vi "try phidget servo.vi"() -> ()   [LabVIEW 2014]
panel:
  in  "Y pos":dbl(slide)=136.3265306122449 scale=120.0..180.0
  out "error out":errorcluster
  in  "X pos":dbl(slide)=107.31292517006803 step=0.1 scale=80.0..135.0 scale format="%#.2g"
  in  "stop":bool
  out "Serial Number Return":i32
  out "Engaged?":bool
  out "Number of\nservos":i32
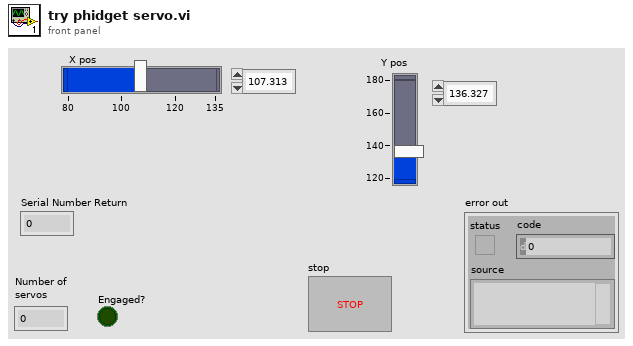
[diagram p1: front panel]
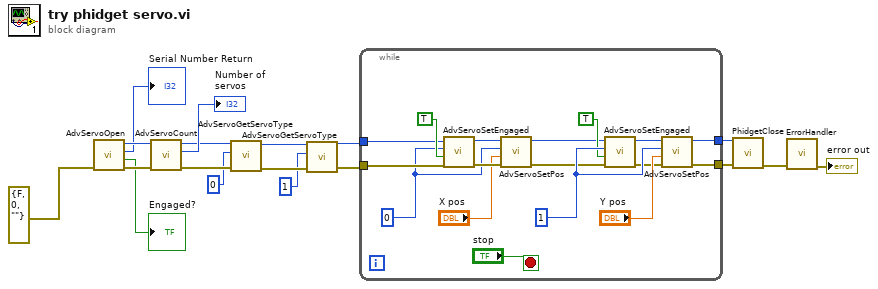
[diagram p0: block diagram]
diagram:
  n1 = call "AdvServoOpen.vi"("error in"=errorcluster {"status"=FALSE, "code"=0, "source"=""} ("error in (no error)")) -> ("error out"=w17:errorcluster, "Attached?"=→"Engaged?":bool, "Serial Number Return"=→"Serial Number Return":i32, "Device Out"=w16:i32)  [unwired: 7 in]
  n2 = call "AdvServoCount.vi"("error in (no error)"=w17, "Device In"=w16) -> ("error out"=w7:errorcluster, "count"=→"Number of\nservos":i32, "Device Out"=w8:i32)  [unwired: 7 in]
  n3 = call "AdvServoGetServoType.vi"("error in (no error)"=w7, "index"=0, "Device In"=w8) -> ("error out"=w4:errorcluster, "Device Out"=w5:i32)  [unwired: 5 in, 1 out]
  n4 = call "AdvServoGetServoType.vi"("error in (no error)"=w4, "index"=1, "Device In"=w5) -> ("error out"=w1:errorcluster, "Device Out"=w2:i32)  [unwired: 5 in, 1 out]
  n5 = while {
    tunnel: w2 -> [w32]
    tunnel: w1 -> [w31]
    tunnel: [w20] -> w10
    tunnel: [w19] -> w9
    stop <- "stop" stop-if-true
    w27 = 1
    w28 = 0
    n6 = call "AdvServoSetEngaged.vi"("error in (no error)"=w31, "SetEngaged"=TRUE, "index"=w28, "Device In"=w32) -> ("error out"=w30:errorcluster, "Device Out"=w33:i32)  [unwired: 5 in]
    n7 = call "AdvServoSetPos.vi"("error in (no error)"=w30, "pos_in"="X pos", "index"=w28, "Device In"=w33) -> ("error out"=w21:errorcluster, "Device Out"=w22:i32)  [unwired: 5 in]
    n8 = call "AdvServoSetEngaged.vi"("error in (no error)"=w21, "SetEngaged"=TRUE, "index"=w27, "Device In"=w22) -> ("error out"=w25:errorcluster, "Device Out"=w24:i32)  [unwired: 5 in]
    n9 = call "AdvServoSetPos.vi"("error in (no error)"=w25, "pos_in"="Y pos", "index"=w27, "Device In"=w24) -> ("error out"=w20:errorcluster, "Device Out"=w19:i32)  [unwired: 5 in]
  }
  n10 = call "PhidgetClose.vi"("error in"=w10, "Device In"=w9) -> ("error out"=w11:errorcluster)  [unwired: 9 in]
  n11 = call "ErrorHandler.vi"("error in"=w11) -> ("error out"=→"error out":errorcluster)  [unwired: 9 in, 1 out]
